vi "presente in tabella si no.vi"(6 "error in (no error)":errorcluster, 8 "colonna":string, 9 "tabella":string, 10 "NOME da cercare":string, 11 "Refnum in":T1) -> (0 "error out":errorcluster, 2 "presente?":bool, 3 "Refnum out":T1)   [LabVIEW 2014]
uses:
  <vilib>/addons/database/Connection.llb/Conn ObjectReference.ctl
  <vilib>/addons/database/_DB Variant To Data/Database Variant To Data.xnode
  <vilib>/addons/database/NI_Database_API.lvlib
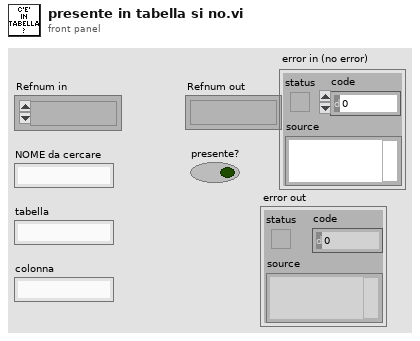
[diagram p1: front panel]
types:
  T1 = typedef "NI_Database_API.lvlib/Conn ObjectReference.ctl" = refnum<k1>
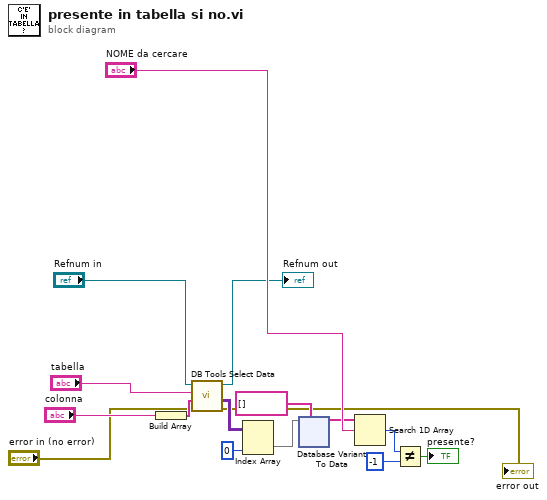
[diagram p0: block diagram]
diagram:
  n1 = Build Array("colonna") -> (w3:string[])
  n2 = call <vilib>:"DB Tools Select Data.vi"("error in (no error)"="error in (no error)", "columns"=w3, "table"="tabella", "connection reference"="Refnum in") -> ("error out"=→"error out":errorcluster, "data"=w9:variant[][], "connection reference out"=→"Refnum out":T1)  [unwired: 2 in]
  n3 = Index Array(array=w9, index (col)=0 ("disabled index (col)")) -> (element=w8:variant[])  [unwired: 1 in]
  n4 = xnode "Database Variant To Data"("database variant"=w8, "type"=string[] []) -> ("data"=w10:string[])  [unwired: 1 in, 1 out]
  n5 = Search 1D Array(1D array=w10, element="NOME da cercare") -> (index of element=w6:i32)  [unwired: 1 in]
  n6 = Not Equal?(x=w6, y=-1) -> (x != y?=→"presente?":bool)
